vi "readDefaultSettings.vi"(8 "error in (no error)":errorcluster, 11 "Model in":refnum<class "Model.lvclass">) -> (0 "error out":errorcluster, 3 "Model out":refnum<class "Model.lvclass">)   [LabVIEW 2015, in "Model.lvclass"]
uses:
  Model.lvclass
  Bootloader/Bootloader.lvclass
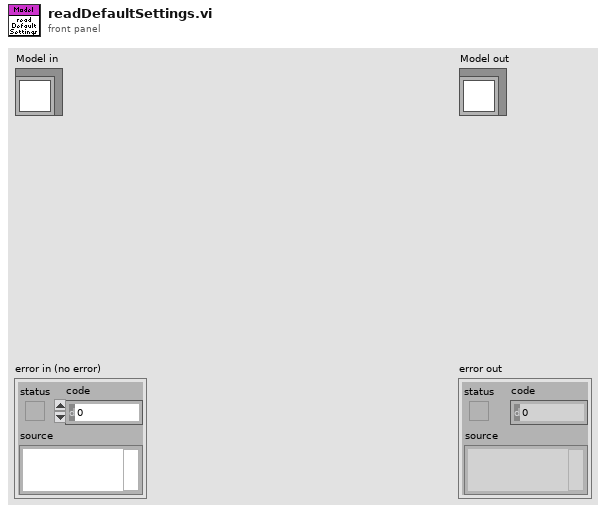
[diagram p1: front panel]
types:
  T1 = typedef "ILCCommon.lvlib/ILCTypedefs.lvlib/Outputs.ctl" = cluster{"Step & Direction":i16, "Blower RPM":u8, "PWM (SSR)":u8, "Ch1":u16, "Ch2":u16, "Ch3":u16, "Ch4":u16}
  T2 = typedef "FAMTTypedefs.lvlib/ForceSensorSettings.ctl" = cluster{"ADC Channel":u8, "Reference Voltage Vref":dbl[unit], "Force Sensor Calculator":T3}
  T3 = typedef "ForceSensorCalculator.lvlib/ForceSensorCalculator.ctl" = cluster{"Capacity":dbl[unit], "Sensitivity":dbl[unit], "Bridge Resistors":T4}
  T4 = typedef "ForceSensorCalculator.lvlib/BridgeResistors.ctl" = cluster{"R1":dbl[unit], "R2":dbl[unit]}
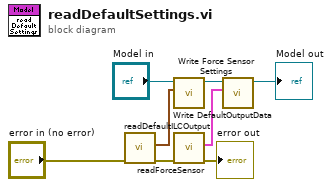
[diagram p0: block diagram]
diagram:
  n1 = call "readDefaultILCOutput.vi"("error in (no error)"="error in (no error)") -> ("error out"=w3:errorcluster, "ILC Outputs"=w7:T1)  [unwired: 8 in, 1 out]
  n2 = call "Write DefaultOutputData.vi"("ILC Outputs"=w7, "Model in"="Model in") -> ("Model out"=w6:refnum<class "Model.lvclass">)  [unwired: 9 in]
  n3 = call "readForceSensor.vi"("error in (no error)"=w3) -> ("error out"=→"error out":errorcluster, "Force Sensor Settings"=w8:T2)  [unwired: 8 in, 1 out]
  n4 = call "Write Force Sensor Settings.vi"("Force Sensor Settings"=w8, "Model in"=w6) -> ("Model out"=→"Model out":refnum<class "Model.lvclass">)  [unwired: 9 in]
